vi "Fault_ID_Parse.vi"(8 "Enum":enum16{"Sequence", "Table"}(ring), 11 "Numeric":u32) -> (3 "String":string)   [LabVIEW 2016]
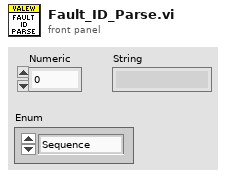
[diagram p1: front panel]
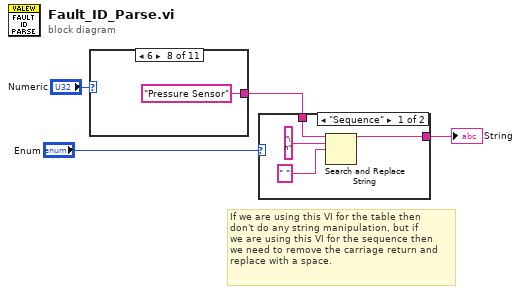
[diagram p0: block diagram]
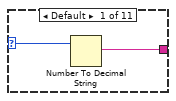
[diagram p3: hidden frame]
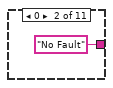
[diagram p4: hidden frame]
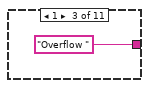
[diagram p5: hidden frame]
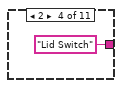
[diagram p6: hidden frame]
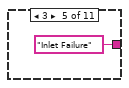
[diagram p7: hidden frame]
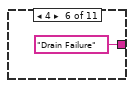
[diagram p8: hidden frame]
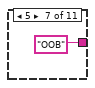
[diagram p9: hidden frame]
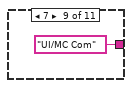
[diagram p10: hidden frame]
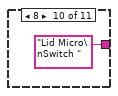
[diagram p11: hidden frame]
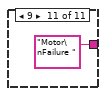
[diagram p12: hidden frame]
diagram:
  # "If we are using this VI for the table then\ndon't do any string manipulation, but if\nwe are using this VI for the sequence then\nwe need to remove the carriage return and\nreplace with a space."
  n1 = case shown="6" "Numeric" {
    selector: "Numeric" -> [w6 _ _ _ _ _ _ _ _ _ _]
    tunnel: [w5 "No Fault" "Overflow " "Lid Switch" "Inlet Failure" "Drain Failure" "OOB" "Pressure Sensor" "UI/MC Com" "Lid Micro\nSwitch " "Motor\nFailure "] -> w3
    frame Default {
      n2 = Number To Decimal String(number=w6) -> (decimal integer string=w5:string)  [unwired: 1 in]
    }
    frame 0 {
    }
    frame 1 {
    }
    frame 2 {
    }
    frame 3 {
    }
    frame 4 {
    }
    frame 5 {
    }
    frame 6 {
    }
    frame 7 {
    }
    frame 8 {
    }
    frame 9 {
    }
  }
  n3 = case shown="\"Sequence\"" "Enum" {
    tunnel: w3 -> [w20 w21]
    tunnel: [w17 w21] -> w2
    frame "Sequence" {
      n4 = Search and Replace String(input string=w20, search string="\n", replace string=" " ("replace string (\"\")")) -> (result string=w17:string)  [unwired: 5 in, 3 out]
    }
    frame "Table" {
    }
  }
  "String" <- w2
